vi "Main-revision2.vi"() -> ()   [LabVIEW 2020]
uses:
  Shared/GUI_Template/TCP subscription info cluster.ctl
  Controls/GUI controls/TabControl--Tab.ctl
  Controls/Loop_data--Cluster.ctl
  Controls/Graph_data--Cluster.ctl
  Controls/GUI controls/GUI_Flags.ctl
  Controls/Database Data.ctl
  Shared/MySQL/typedefs/mysql_authentication.ctl
  <userlib>/_OpenG.lib/array/array.llb/Filter 1D Array with Scalar (String)__ogtk.vi
  Shared/MySQL/Preset Query Enum.ctl
panel:
  out "TCP subscriptions info":T1
  out "StopQueue":refnum<queue>
  out "DataQueue":refnum<queue>
  out "error out":errorcluster
  out "error TCP Open":errorcluster
  out "error TCP  Write":errorcluster
  in  "Tab Control":enum32{"Home", "Settings", "Plot", "Save"}(tab)
  in  "Database Variable List":i32[](listbox)
  in  "Plotter ID (Simulate)":string
  out "Query":string
  in  "Add variables":bool
  out "Long Term Plot":cluster{timestamp[], dbl[]}[](graph)
  in  "Clear Graph":bool
  out "short Term Plot":cluster{timestamp[], dbl[]}[](graph) caption="Long Term Plot"
  in  "Stop":bool
  in  "Simulate":bool
  out "Data read by TCP":string[](array[string])
  out "appargs 2":string[](array[string])
  out "min Left":i16
  out "min Top":i16
  out "max Right":i16
  out "max Bottom":i16
  in  "Read INI File":bool
  in  "Configuration File Path":path=path "C:/Users/Priyanka/Documents/Plotter/Data/Plot Configuration.txt"
  out "Subscribe commands":string[](array[string])=["Wait>>Exposure,Gain", "Wait>>Exposure"]
  out "IP Addresses of interested  devices":string[](array[string])
  out "appended array":string[][](array[string])
  in  "reference out":refnum<vi>
  out "time to open ref":u32
  out "Device Infor from Database":string[][](array[string])
  in  "Plot":bool=TRUE
  in  "Settings":bool
  in  "Home":bool
  # "Settings"
  # "Plot"
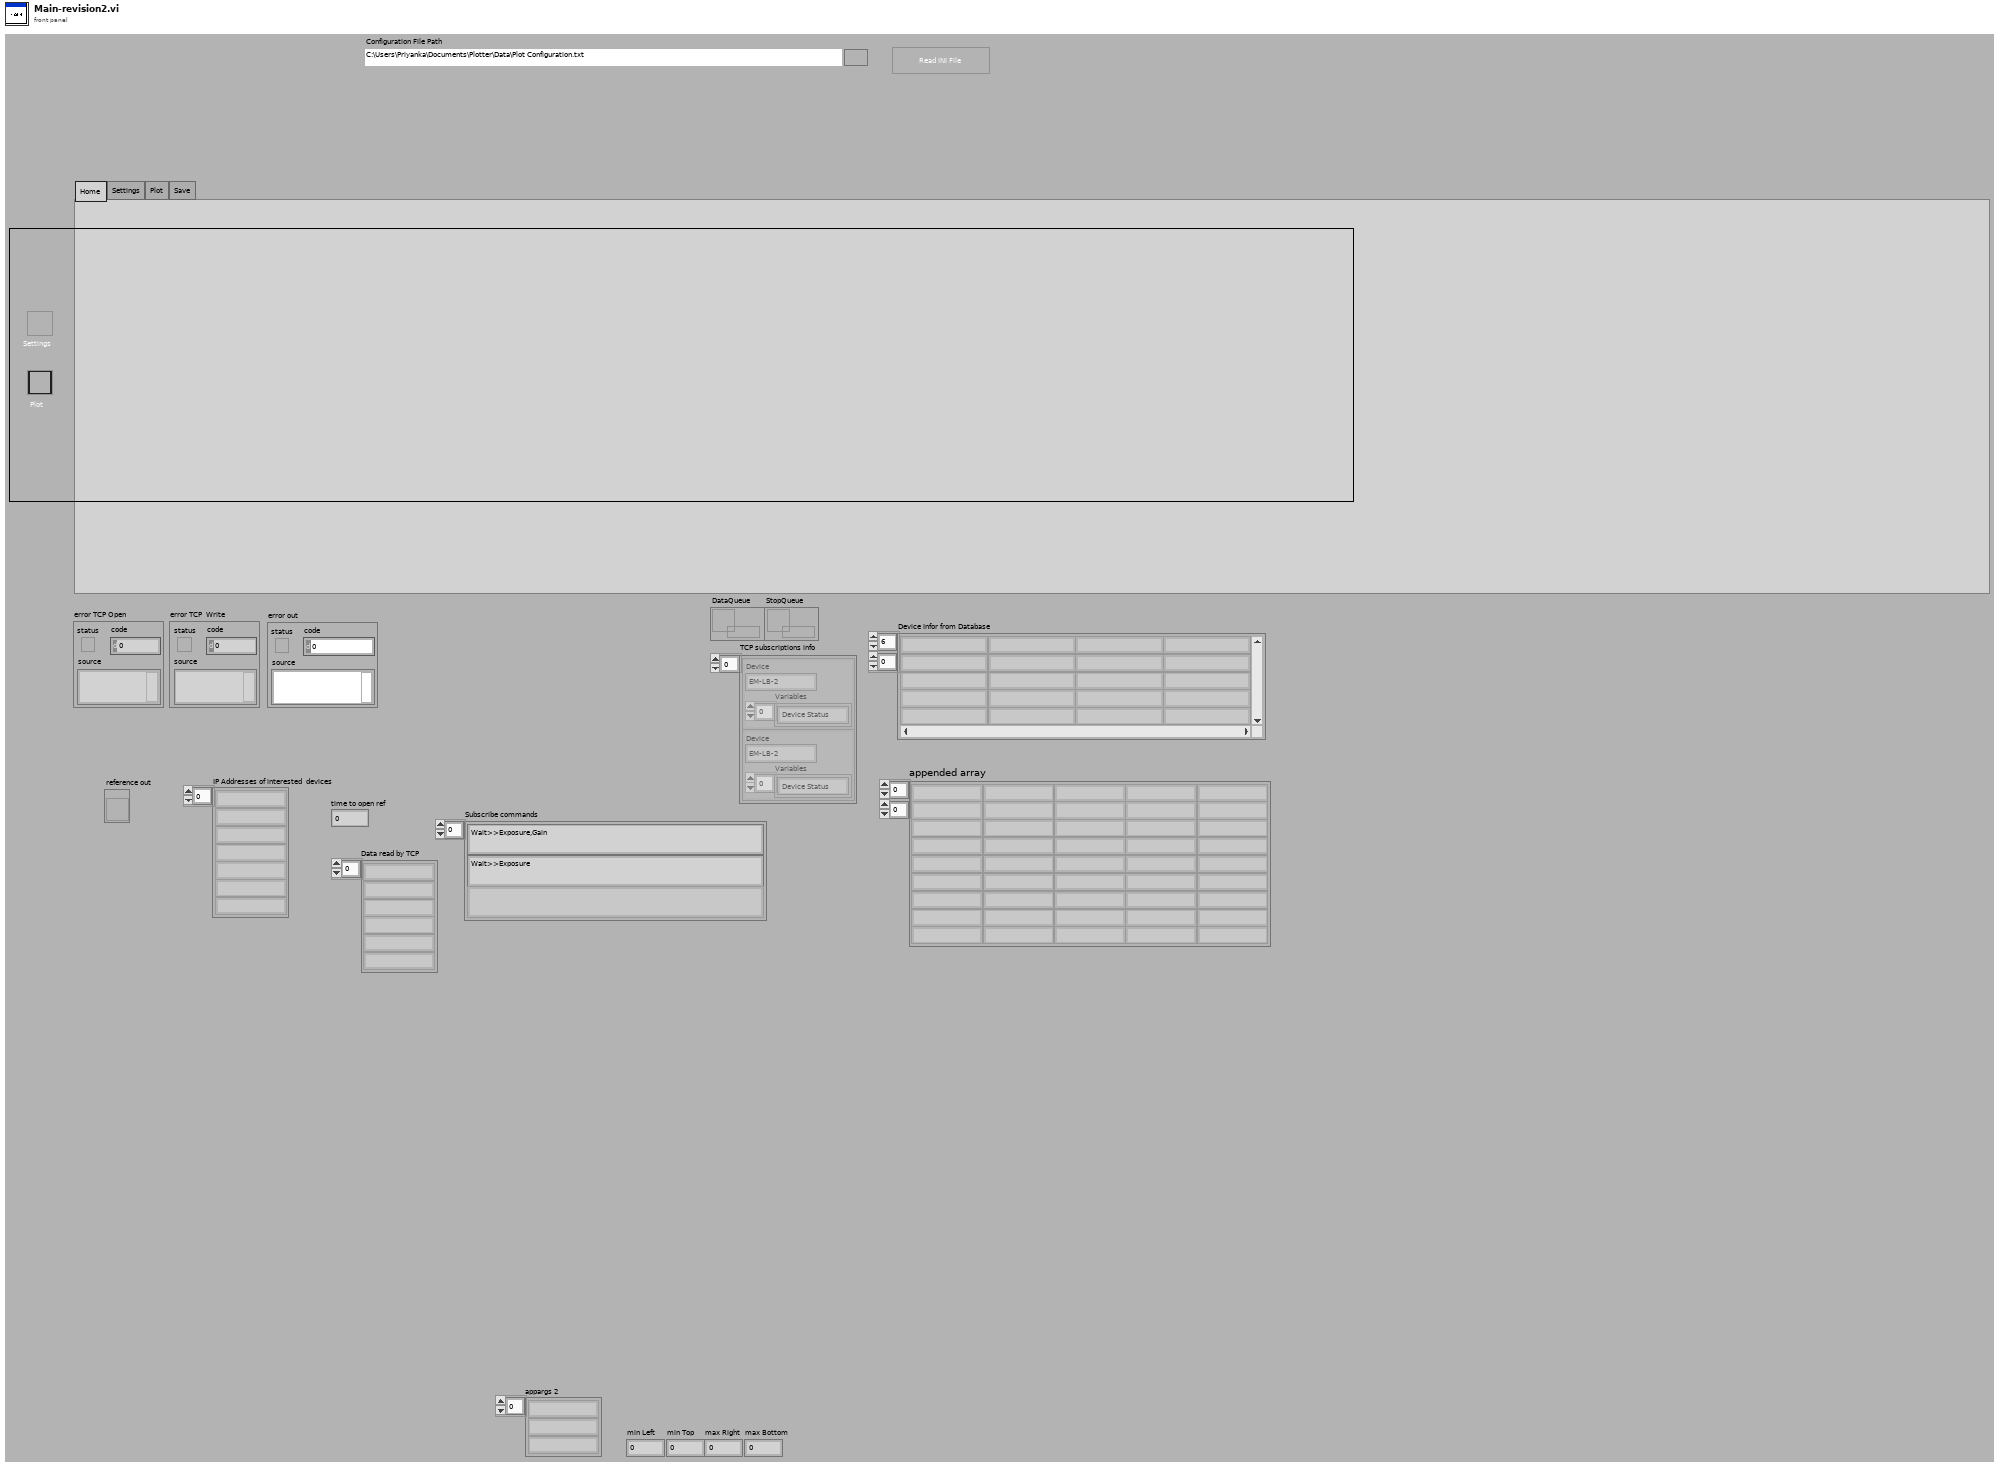
[diagram p1: front panel]
types:
  T1 = typedef "TCP subscription info cluster.ctl" = cluster{"Device":string, "Variables":string[]}[]
  T2 = typedef "LVAllMonitorsDisplayTypeDef.ctl" = cluster{"Bounds":cluster{"Left":i16, "Top":i16, "Right":i16, "Bottom":i16}, "Depth":i16}[]
  T3 = typedef "TabControl--Tab.ctl" = enum32{"Home", "Settings", "Plot", "Save"}
  T4 = cluster{"Selected Variables":string[][], "Data.TCP ports":refnum<k5>[]}
  T5 = enum32{"invalid app kind", "Development System", "Run Time System", "Student Edition", "Embedded LabVIEW", "Evaluation", "Custom"}
  T6 = typedef "Preset Query Enum.ctl" = enum16{"Get Locations", "Get all IPs and MACs", "Get classes", "Get expt variables to set at scanstart for particular device", "Get expt devices and variables with start values", "Get expt devices and variables (with data to get)", "Get expt devices with data to get", "Get Expt devices and GUIs", "Get all devices basic properties", "Get Virtual Devices Core Info", "Get Expt names", "Get experiment basic properties", "Get experiment alarm variables", "Get MC Ports", "Get device network comm port", "Get devicetype lvclass path", "Get basic device properties", "Get Init Order", "Get all setable variables of a device", "Get device variable aliases", "Get force values of all settable variables", "Get all variables of a devicetype", "Get all variables of a device", "Get plotter details", "Get Saved Scans", "Get Scan Info", "GetGeneralGUIs", "Get expt for plotter", "Get plotter IDs from expt", "Get all devices", "Get all Virtual Devices", "Get all aliases", "Get variable and device info for Virtual Device", "GetItemLocatorIP", "Get IPs for GUIs", "Get DeviceType from Device", "GetLocalPortRange", "GetDevicePresetVariables", "Get Device Configuration", "GetAllPresetNames", "GetAllConfigurationNames", "GetPresetDeviceNames", "GetDeviceAliases", "GetDevicesOfClass"}
  T7 = enum32{"Invalid", "Standard", "Closed", "Hidden", "Minimized", "Maximized"}
  T8 = typedef "Loop_data--Cluster.ctl" = cluster{"INI Data":string[][], "Currently selected items":i32[], "Selected Variables":string[][], "No of Selected Variables":i32, "Data":dbl[], "Simulate":bool, "Start":bool, "Legend Rows":i32, "Init":bool}
  T9 = typedef "Graph_data--Cluster.ctl" = cluster{"Graph Data Long":cluster{"Timestamp":timestamp[], "Data Array":dbl[]}[], "Graph Data Short":cluster{"Timestamp":timestamp[], "Data Array":dbl[]}[], "Short term plot":refnum<vi>, "Long term plot ":refnum<vi>, "ms timer value":u32}
  T10 = typedef "GUI_Flags.ctl" = cluster{"Start":bool, "Stop":bool, "Read INI File":bool, "Tab Control":enum32{"Home", "Settings", "Plot", "Save"}, "Settings":bool, "Home":bool, "Plot":bool}
  T11 = typedef "Database Data.ctl" = cluster{"SQL Server Info":cluster{"Port":u16, "IP Address":string, "Authentication":T12}, "Variables":string[], "Devices":string[], "Display Names (for variables)":string[], "Variable Data ID":string, "Variable display info":string[][], "Plotter ID":string, "Device space Variable":string[]}
  T12 = typedef "mysql_authentication.ctl" = cluster{"User":string, "Password":string, "Database":string}
  T13 = cluster{"Core":cluster{"Current VI Reference":refnum<vi>, "Close Panel on Exit?":bool}, "Data":T8, "Graph":T9, "reference out":refnum<vi>, "GUI controls":T10, "Database Data":T11, "TCP ports":refnum<k5>[]}
  T14 = cluster{"Current VI Reference":refnum<vi>, "Close Panel on Exit?":bool}
  T15 = cluster{"Port":u16, "IP Address":string, "Authentication":T12}
  T16 = cluster{"Timestamp":timestamp[], "Data Array":dbl[]}[]
  T17 = cluster{"Any timeouts?":bool, "tcp read times":u32[], "Errors":errorcluster[], "tcp Data parsed array":string[][]}
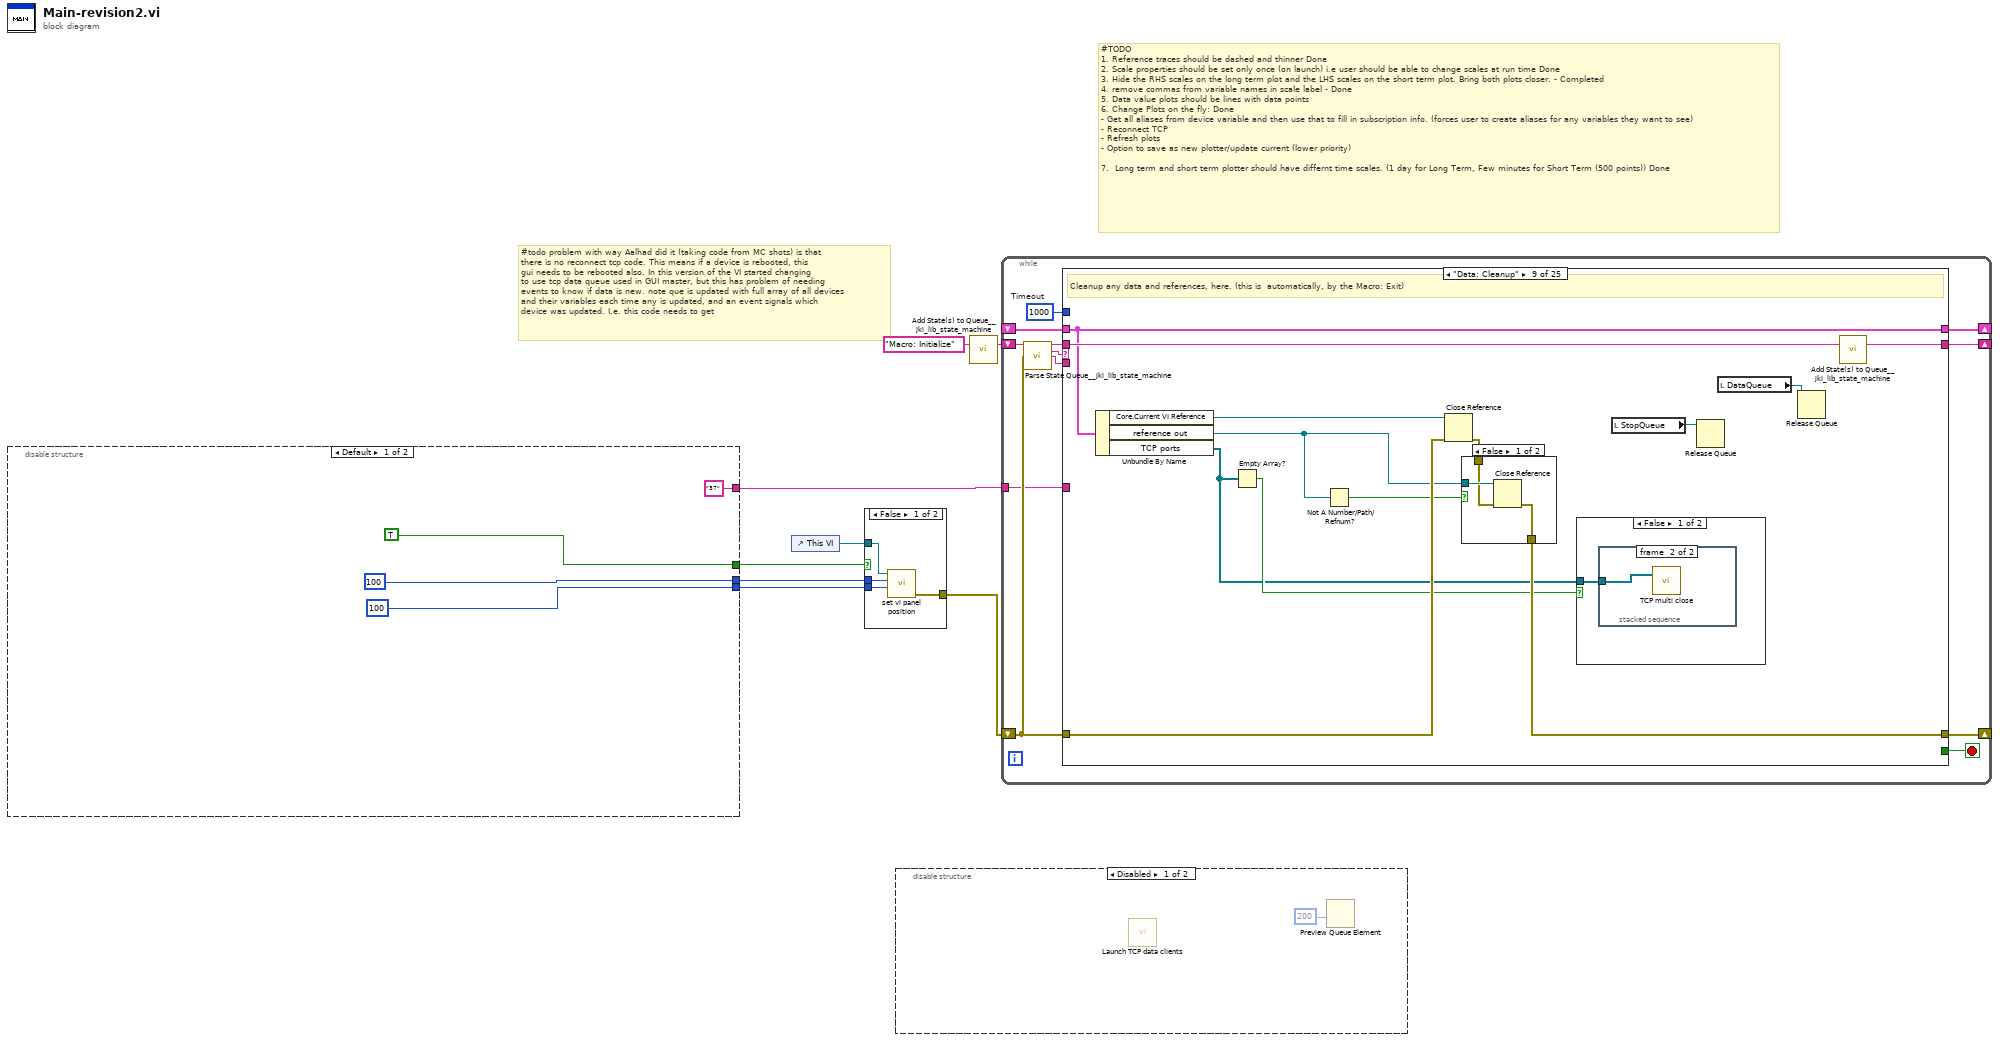
[diagram p0: block diagram]
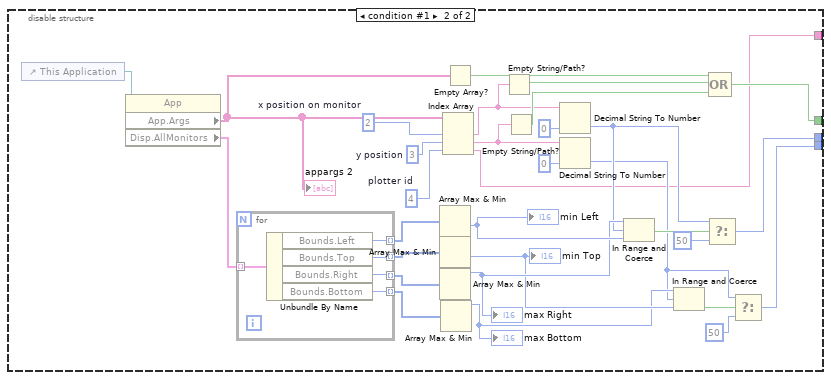
[diagram p4: hidden frame]
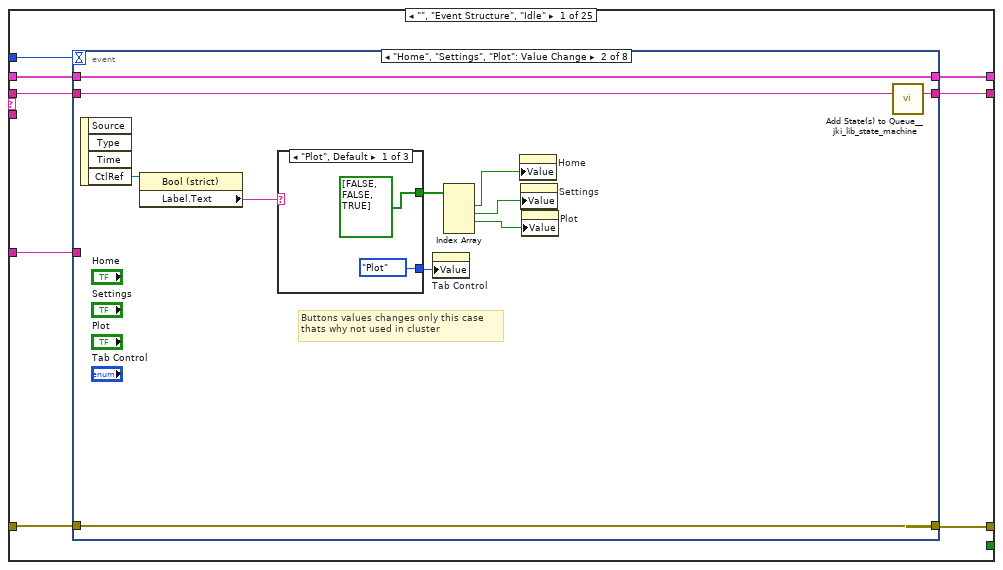
[diagram p5: hidden frame]
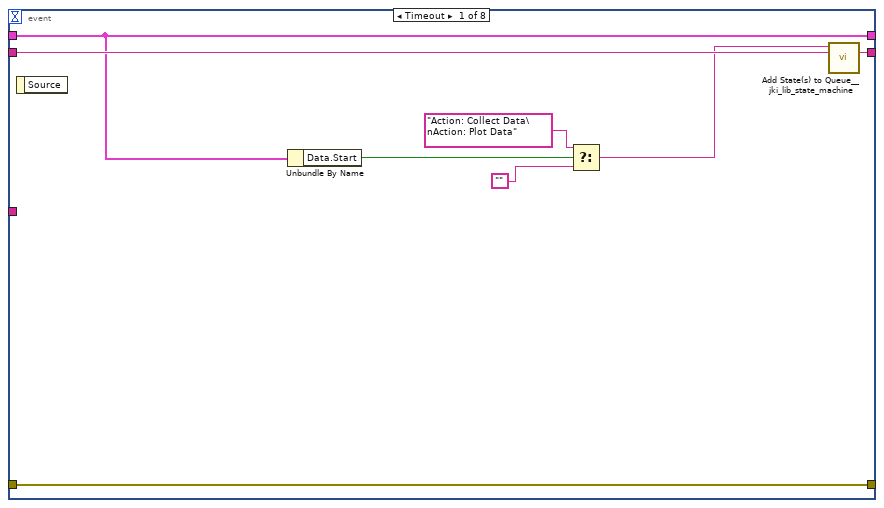
[diagram p6: hidden frame]
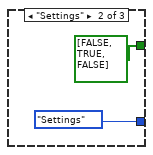
[diagram p7: hidden frame]
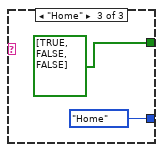
[diagram p8: hidden frame]
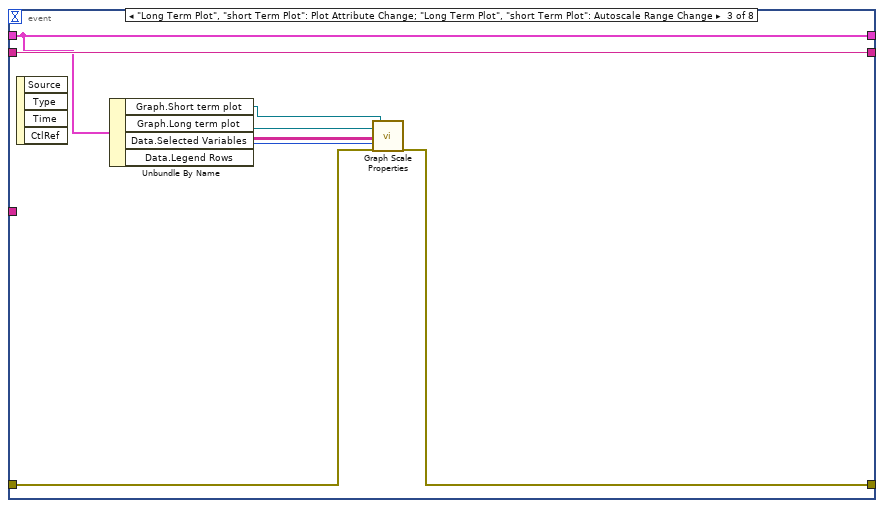
[diagram p9: hidden frame]
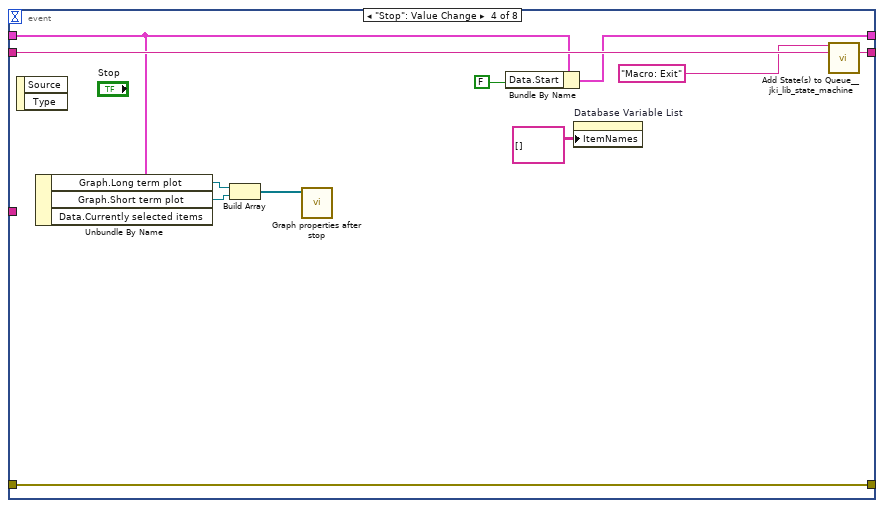
[diagram p10: hidden frame]
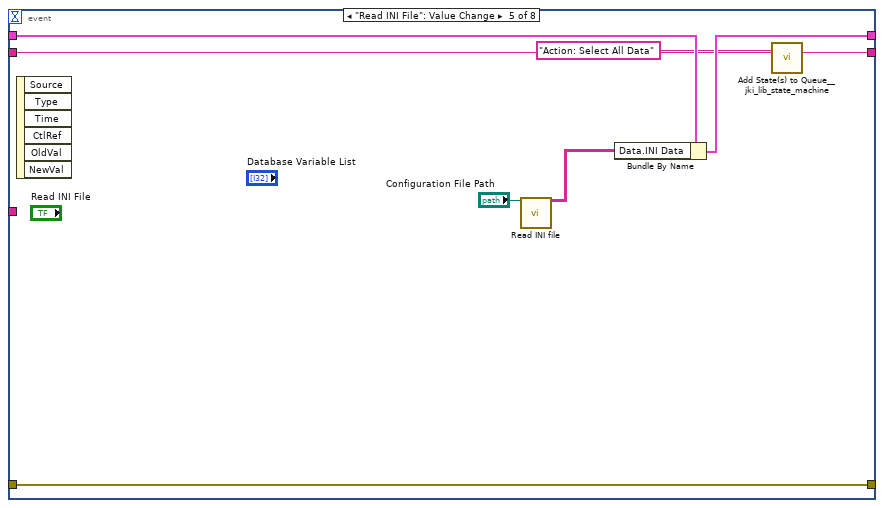
[diagram p11: hidden frame]
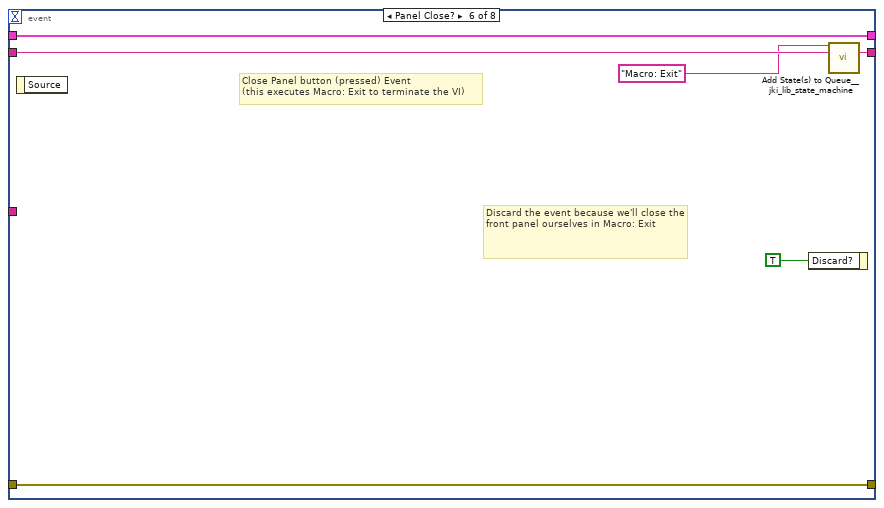
[diagram p12: hidden frame]
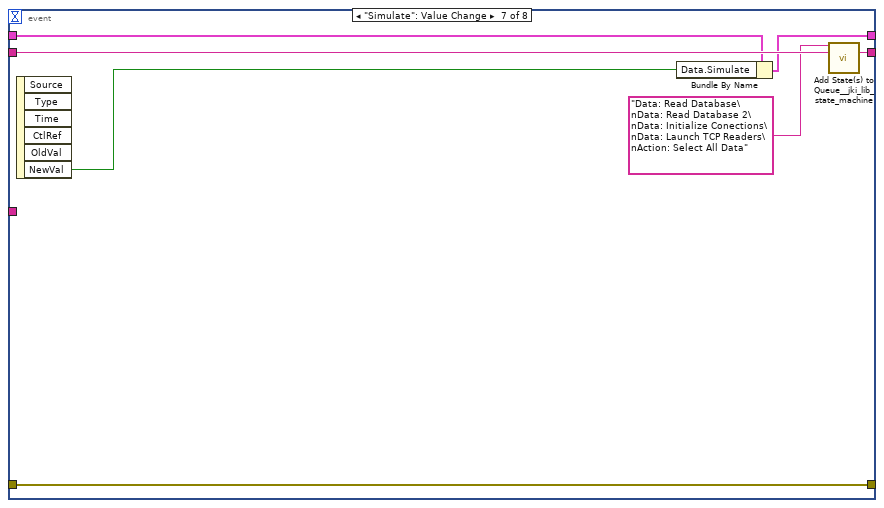
[diagram p13: hidden frame]
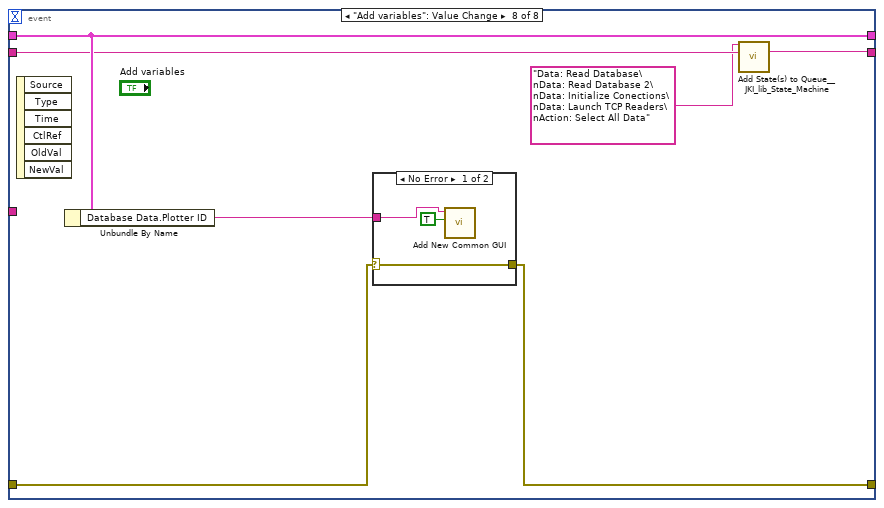
[diagram p14: hidden frame]
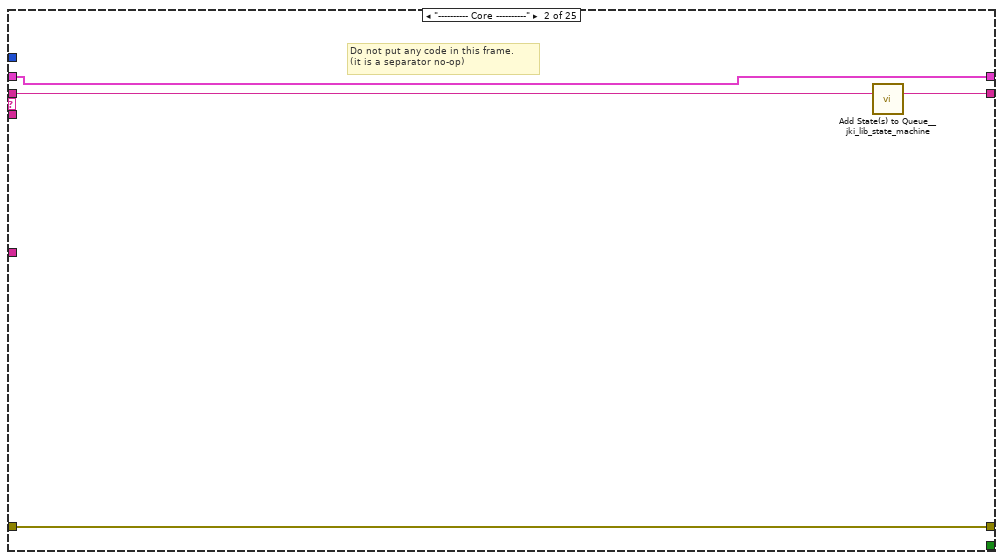
[diagram p16: hidden frame]
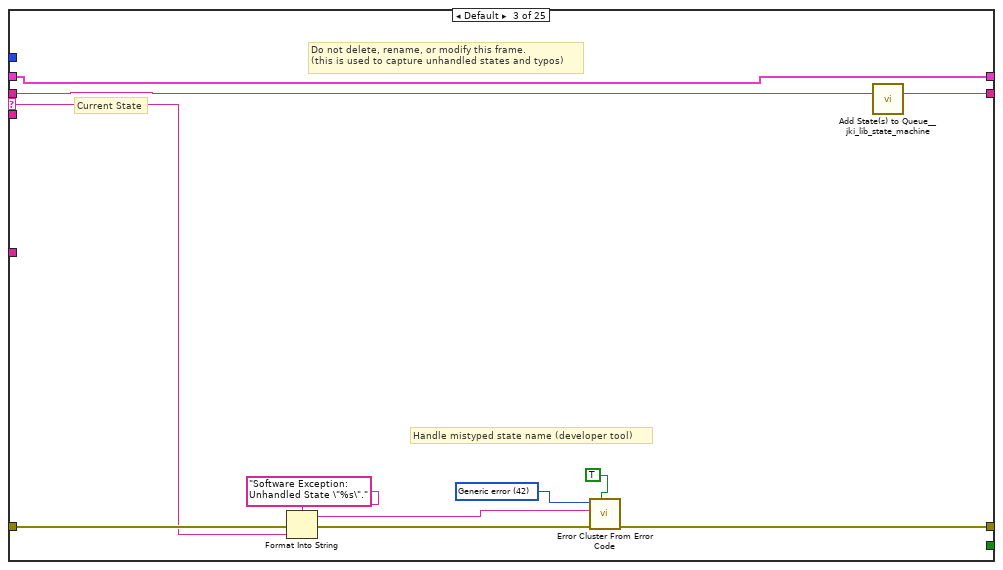
[diagram p17: hidden frame]
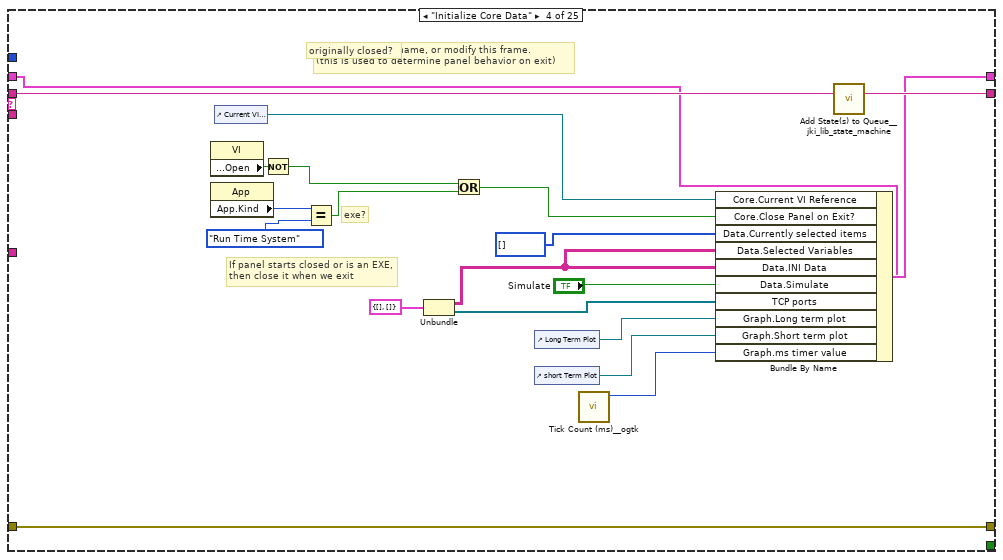
[diagram p18: hidden frame]
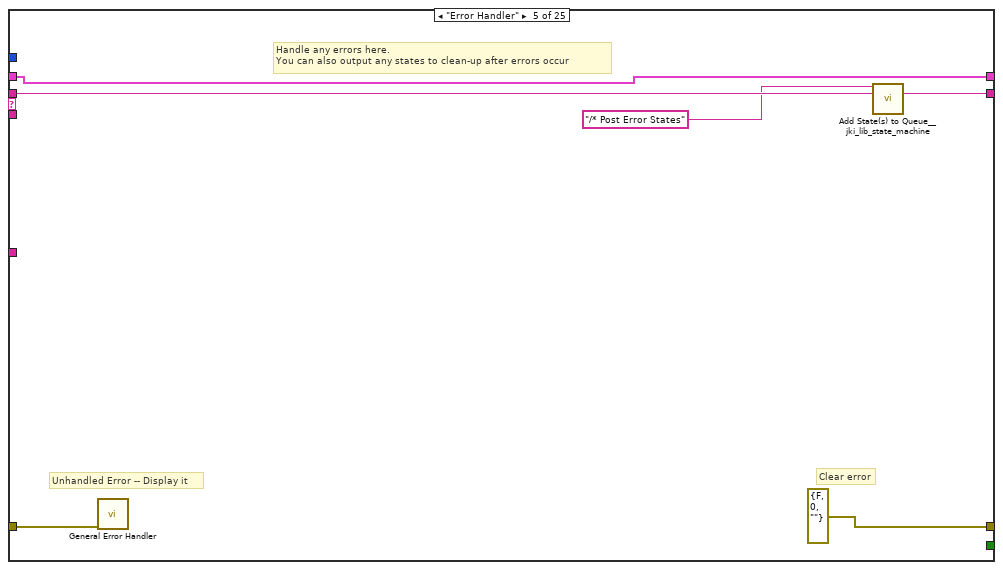
[diagram p19: hidden frame]
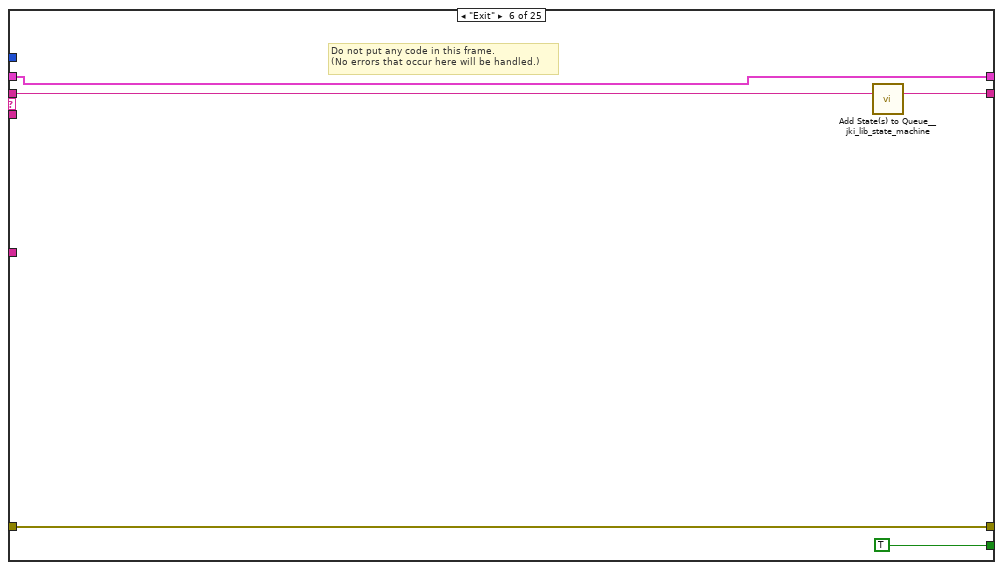
[diagram p20: hidden frame]
diagram:
  # "#todo problem with way Aalhad did it (taking code from MC shots) is that\nthere is no reconnect tcp code. This means if a device is rebooted, this\ngui needs to be rebooted also. In this version of the VI started changing\nto use tcp data queue used in GUI master, but this has problem of needing\nevents to know if data is new. note que is updated with full array of all devices\nand their variables each time any is updated, and an event signals which\ndevice was updated. I.e. this code needs to get"
  # "#TODO\n1. Reference traces should be dashed and thinner Done\n2. Scale properties should be set only once (on launch) i.e user should be able to change scales at run time Done\n3. Hide the RHS scales on the long term plot and the LHS scales on the short term plot. Bring both plots closer. - Completed\n4. remove commas from variable names in scale label - Done \n5. Data value plots should be lines with data points\n6. Change Plots on the fly: Done\n- Get all aliases from device variable and then use that to fill in subscription info. (forces user to create aliases for any variables they want to see)\n- Reconnect TCP\n- Refresh plots\n- Option to save as new plotter/update current (lower priority)\n\n7.  Long term and short term plotter should have differnt time scales. (1 day for Long Term, Few minutes for Short Term (500 points)) Done"
  n1 = disable-structure shown="Default" {
    disable-tunnel: [100 ("number") w27] -> w4
    disable-tunnel: [100 ("number") w22] -> w5
    disable-tunnel: [TRUE w17] -> w6
    disable-tunnel: ["37" w14] -> w1
    frame condition #0 (active) {
    }
    frame condition #1 {
      w15 = 4  # plotter id
      w42 = 3  # y position
      w43 = 2  # x position on monitor
      n2 = control-ref of="This Application"() -> (w16:refnum<vi>)
      n3 = property class="App"(reference=w16) -> ("App.Args"=w41:string[], "Disp.AllMonitors"=w36:T2)  [unwired: 1 in, 2 out]
      "appargs 2" <- w41
      n4 = for {
        tunnel: w36 -> [w48] mode=indexing
        tunnel: [w47] -> w37 mode=indexing
        tunnel: [w46] -> w38 mode=indexing
        tunnel: [w45] -> w39 mode=indexing
        tunnel: [w44] -> w40 mode=indexing
        n5 = Unbundle By Name(w48) -> ("Bounds.Left"=w47:i16, "Bounds.Top"=w46:i16, "Bounds.Right"=w45:i16, "Bounds.Bottom"=w44:i16)
      }
      n6 = Array Max & Min(array=w37) -> (min value=w35:i16)  [unwired: 3 out]
      "min Left" <- w35
      n7 = Array Max & Min(array=w38) -> (min value=w33:i16)  [unwired: 3 out]
      "min Top" <- w33
      n8 = Array Max & Min(array=w39) -> (max value=w34:i16)  [unwired: 3 out]
      "max Right" <- w34
      n9 = Array Max & Min(array=w40) -> (max value=w32:i16)  [unwired: 3 out]
      "max Bottom" <- w32
      n10 = Index Array(array=w41, index #1=w43, index #2=w42, index #3=w15) -> (element #1=w13:string, element #2=w21:string, element #3=w14:string)
      n11 = Empty Array?(array=w41) -> (empty?=w20:bool)
      n12 = Empty String/Path?(string/path=w13) -> (empty?=w19:bool)
      n13 = Empty String/Path?(string/path=w21) -> (empty?=w18:bool)
      n14 = Decimal String To Number(string=w13, default (0L)=i16 0 ("default (0 I32)")) -> (number=w28:i16)  [unwired: 1 in, 1 out]
      n15 = Decimal String To Number(string=w21, default (0L)=i16 0 ("default (0 I32)")) -> (number=w23:i16)  [unwired: 1 in, 1 out]
      n16 = In Range and Coerce(upper limit=w34, x=w28, lower limit=w35) -> (In Range?=w29:bool)  [unwired: 1 out]
      n17 = In Range and Coerce(upper limit=w32, x=w23, lower limit=w33) -> (In Range?=w24:bool)  [unwired: 1 out]
      n18 = Select(t=w28, s=w29, f=i16 50) -> (s? t:f=w27:i16)
      n19 = Compound Arithmetic op=OR(w20, w19, w18) -> (w17:bool)
      n20 = Select(t=w23, s=w24, f=i16 50) -> (s? t:f=w22:i16)
    }
  }
  n21 = control-ref of="This VI"() -> (w3:refnum<vi>)
  n22 = case shown="False" w6 {
    tunnel: w4 -> [w52 _]
    tunnel: w5 -> [w51 _]
    tunnel: w3 -> [w50 _]
    tunnel: [w49 _] -> w2
    frame False {
      n23 = call "set vi panel position.vi"("top"=w51, "left"=w52, "This VI"=w50) -> ("error out"=w49:errorcluster)  [unwired: 7 in, 1 out]
    }
    frame True {
    }
  }
  n24 = disable-structure shown="Disabled" {
    frame Disabled {
      n25 = call "Launch TCP data clients.vi"() -> ()  [unwired: 10 in, 2 out]
      n26 = Preview Queue Element(timeout in ms (-1)=200) -> ()  [unwired: 2 in, 4 out]
    }
    frame Enabled {
    }
  }
  n27 = call <vilib>:"Add State(s) to Queue__jki_lib_state_machine.vi"("State(s) in (\"\")"="Macro: Initialize") -> ("States Out"=w8:string)  [unwired: 14 in]
  n28 = while {
    shift-right: [w59] -> _
    shift-left: _ -> [w58]
    shift-right: [w62] -> _
    shift-left: w2 -> [w56]
    shift-right: [w61] -> _
    shift-left: w8 -> [w63]
    tunnel: w1 -> [w54]
    stop <- w60 stop-if-true
    w57 = 1000  # Timeout
    n29 = call <vilib>:"Parse State Queue__jki_lib_state_machine.vi"("State Queue"=w63, "Error In (no error)"=w56) -> ("Remaining States"=w65:string, "Current State"=w55:string, "Arguments"=w64:string)  [unwired: 11 in]
    n30 = case shown="\"Data: Cleanup\"" w55 {
      selector: w55 -> [_ _ w154 _ _ _ _ _ _ _ _ _ _ _ _ _ _ _ _ _ _ _ _ _ _]
      tunnel: w65 -> [w73 w153 w158 w184 w190 w195 w199 w210 w223 w252 w285 w299 w335 w371 w381 w387 w398 w424 w431 w441 w445 w449 w481 w507 w557]
      tunnel: w64 -> [_ _ _ _ _ _ _ _ _ _ _ _ _ _ _ w382 w392 _ _ _ _ _ _ _ _]
      tunnel: w58 -> [w71 w150 w156 w175 w187 w193 w196 _ w219 w237 w279 w296 w329 w368 w372 w385 w394 w421 w426 w438 w442 w451 w476 w501 w553]
      tunnel: [w70 w151 w160 w181 errorcluster {"status"=FALSE, "code"=0, "source"=""} ("error out") w192 w197 w207 w217 w250 w282 w291 w330 w369 w379 w383 w395 w422 w428 w439 w443 w457 w479 w502 w549] -> w62
      tunnel: w56 -> [w69 w151 w159 w181 w186 w192 w197 w207 w220 w250 w283 w292 w331 w369 w379 w384 w396 w422 w429 w439 w443 w457 w479 w503 w541]
      tunnel: [w72 w152 w157 w183 w189 w194 w198 w209 w222 w251 w284 w298 w334 w370 w380 w386 w397 w423 w430 w440 w444 w448 w480 w506 w556] -> w61
      tunnel: [_ _ _ _ _ TRUE _ _ _ _ _ _ _ _ _ _ _ _ _ _ _ _ _ _ _] -> w60
      tunnel: [w68 w150 w156 w182 w187 w193 w196 w208 w219 w249 w281 w295 w327 w368 w372 w385 w394 w421 w426 w438 w442 w450 w477 w500 w555] -> w59
      tunnel: w57 -> [w67 _ _ _ _ _ _ _ _ _ _ _ _ _ _ _ _ _ _ _ _ _ _ _ _]
      tunnel: w54 -> [w66 _ _ _ _ _ _ _ _ w234 _ _ _ _ _ _ _ _ _ _ _ _ _ _ _]
      frame "", "Event Structure", "Idle" {
        n31 = event shown="[1] \"Home\", \"Settings\", \"Plot\": Value Change" {
          selector: _ -> [_ _ _ _ _ _ _ _]
          dyn-events: _ -> [_ _ _ _ _ _ _ _]
          timeout: w67 -> [_ _ _ _ _ _ _ _]
          tunnel: w73 -> [w81 w92 w106 w117 w120 w131 w138 w143]
          tunnel: [w80 w91 w106 w116 w119 w130 w137 w142] -> w72
          tunnel: w71 -> [w77 w86 w105 w111 w122 w128 w135 w145]
          tunnel: [w79 w90 w101 w115 w125 w129 w136 w139] -> w70
          tunnel: w69 -> [w79 w90 w102 w115 w125 w129 w136 w140]
          tunnel: [w77 w86 w105 w113 w121 w128 w134 w145] -> w68
          tunnel: w66 -> [_ _ _ _ _ _ _ _]
          event Timeout {
            n32 = event-data() -> ()  [unwired: 1 in, 1 out]
            n33 = Unbundle By Name(w77) -> ("Data.Start"=w76:bool)
            n34 = Select(t="Action: Collect Data\nAction: Plot Data" ("f"), s=w76, f="") -> (s? t:f=w78:string)
            n35 = call <vilib>:"Add State(s) to Queue__jki_lib_state_machine.vi"("State(s) in Front (\"\")"=w78, "State(s) in (\"\")"=w81) -> ("States Out"=w80:string)  [unwired: 13 in]
          }
          event "Home", "Settings", "Plot": Value Change {
            # "Buttons values changes only this case \nthats why not used in cluster"
            n36 = event-data() -> ("CtlRef"=w89:refnum<vi>)  [unwired: 1 in, 3 out]
            n37 = property class="Bool (strict)"(reference=w89) -> ("Label.Text"=w88:string)  [unwired: 1 in, 2 out]
            n38 = case shown="\"Plot\", Default" w88 {
              tunnel: [TabControl--Tab."Plot" ("Tab Control") TabControl--Tab."Settings" ("Tab Control") TabControl--Tab."Home" ("Tab Control")] -> w82
              tunnel: [bool[] [FALSE, FALSE, TRUE] bool[] [FALSE, TRUE, FALSE] bool[] [TRUE, FALSE, FALSE]] -> w87
              frame "Plot", Default {
              }
              frame "Settings" {
              }
              frame "Home" {
              }
            }
            n39 = property on="Tab Control" class="TabCtl (strict)"("Value"=w82) -> ()  [unwired: 2 in, 2 out]
            n40 = Index Array(array=w87) -> (element #1=w85:bool, element #2=w84:bool, element #3=w83:bool)  [unwired: 4 in, 1 out]
            n41 = property on="Home" class="Bool (strict)"("Value"=w85) -> ()  [unwired: 2 in, 2 out]
            n42 = property on="Settings" class="Bool (strict)"("Value"=w84) -> ()  [unwired: 2 in, 2 out]
            n43 = property on="Plot" class="Bool (strict)"("Value"=w83) -> ()  [unwired: 2 in, 2 out]
            n44 = call <vilib>:"Add State(s) to Queue__jki_lib_state_machine.vi"("State(s) in (\"\")"=w92) -> ("States Out"=w91:string)  [unwired: 14 in]
          }
          event "Long Term Plot", "short Term Plot": Plot Attribute Change; "Long Term Plot", "short Term Plot": Autoscale Range Change {
            n45 = event-data() -> ()  [unwired: 1 in, 4 out]
            n46 = Unbundle By Name(w105) -> ("Graph.Short term plot"=w103:refnum<vi>, "Graph.Long term plot"=w99:refnum<vi>, "Data.Selected Variables"=w104:string[][], "Data.Legend Rows"=w100:i32)
            n47 = call "Graph Scale Properties.vi"("Long term plot"=w99, "Selected Variables"=w104, "Legend Rows"=w100, "error in (no error)"=w102, "Short term graph"=w103) -> ("error out"=w101:errorcluster)  [unwired: 14 in]
          }
          event "Stop": Value Change {
            n48 = event-data() -> ()  [unwired: 1 in, 2 out]
            n49 = Unbundle By Name(w111) -> ("Graph.Long term plot"=w108:refnum<vi>, "Graph.Short term plot"=w107:refnum<vi>)  [unwired: 1 out]
            n50 = Build Array(w108, w107) -> (w109:refnum<vi>[])
            n51 = call "Graph properties after stop.vi"("Array"=w109) -> ()  [unwired: 11 in]
            n52 = Bundle By Name(cluster=w111, "Data.Start"=FALSE) -> (w113:T13)
            n53 = property on="Database Variable List" class="MCListbox (strict)"("ItemNames"=string[][] [] ("Item Names")) -> ()  [unwired: 2 in, 2 out]
            n54 = call <vilib>:"Add State(s) to Queue__jki_lib_state_machine.vi"("State(s) in Front (\"\")"="Macro: Exit", "State(s) in (\"\")"=w117) -> ("States Out"=w116:string)  [unwired: 13 in]
          }
          event "Read INI File": Value Change {
            n55 = event-data() -> ()  [unwired: 1 in, 6 out]
            n56 = call "Read INI file.vi"("Path"="Configuration File Path") -> ("Data"=w123:string[][])  [unwired: 9 in, 5 out]
            n57 = Bundle By Name(cluster=w122, "Data.INI Data"=w123) -> (w121:T13)
            n58 = call <vilib>:"Add State(s) to Queue__jki_lib_state_machine.vi"("State(s) in Front (\"\")"="Action: Select All Data" ("State(s) in Front (\"\")"), "State(s) in (\"\")"=w120) -> ("States Out"=w119:string)  [unwired: 13 in]
          }
          event Panel Close? {
            # "Discard the event because we'll close the front panel ourselves in Macro: Exit"
            # "Close Panel button (pressed) Event\n(this executes Macro: Exit to terminate the VI)"
            n59 = event-data() -> ()  [unwired: 1 in, 1 out]
            n60 = event-data("Discard?"=TRUE) -> ()  [unwired: 1 in, 1 out]
            n61 = call <vilib>:"Add State(s) to Queue__jki_lib_state_machine.vi"("State(s) in Front (\"\")"="Macro: Exit", "State(s) in (\"\")"=w131) -> ("States Out"=w130:string)  [unwired: 13 in]
          }
          event "Simulate": Value Change {
            n62 = event-data() -> ("NewVal"=w133:bool)  [unwired: 1 in, 5 out]
            n63 = Bundle By Name(cluster=w135, "Data.Simulate"=w133) -> (w134:T13)
            n64 = call <vilib>:"Add State(s) to Queue__jki_lib_state_machine.vi"("State(s) in Front (\"\")"="Data: Read Database\nData: Read Database 2\nData: Initialize Conections\nData: Launch TCP Readers\nAction: Select All Data" ("State(s) in Front (\"\")"), "State(s) in (\"\")"=w138) -> ("States Out"=w137:string)  [unwired: 13 in]
          }
          event "Add variables": Value Change {
            n65 = event-data() -> ()  [unwired: 1 in, 6 out]
            n66 = Unbundle By Name(w145) -> ("Database Data.Plotter ID"=w144:string)
            n67 = case shown="No Error" w140 {
              selector: w140 -> [w146 w149]
              tunnel: w144 -> [w147 _]
              tunnel: [w146 w149] -> w139
              frame No Error {
                n68 = call "Add New Common GUI.vi"("With Alias"=TRUE, "Plotter ID"=w147) -> ()  [unwired: 10 in]
              }
              frame Error {
              }
            }
            n69 = call <vilib>:"Add State(s) to Queue__JKI_lib_State_Machine.vi"("State(s) in Front (\"\")"="Data: Read Database\nData: Read Database 2\nData: Initialize Conections\nData: Launch TCP Readers\nAction: Select All Data", "State(s) in (\"\")"=w143) -> ("States Out"=w142:string)  [unwired: 13 in]
          }
        }
      }
      frame "---------- Core ----------" {
        # "Do not put any code in this frame.\n(it is a separator no-op)"
        n70 = call <vilib>:"Add State(s) to Queue__jki_lib_state_machine.vi"("State(s) in (\"\")"=w153) -> ("States Out"=w152:string)  [unwired: 14 in]
      }
      frame Default {
        w163 = 42 items=["No error", "Argument error", "Memory is full", "Out of zone", "End of file", "File already open", "Generic file I/O error", "File not found", "File permission error", "Disk is full", "Duplicate path", "Too many files open", "System feature not enabled", "Resource file not found", "Cannot add resource", "Resource not found", "Image not found", "Image memory error", "Pen does not exist", "Config type invalid", "Config token not found", "Config parse error", "Config memory error", "Bad external code format", "Bad external code offset", "External code not present", "Null window", "Destroy window error", "Null menu", "Print aborted", "Bad print record", "Print driver error", "Windows error during printing", "Memory error during printing", "Print dialog error", "Generic print error", "Invalid device refnum", "Device not found", "Device parameter error", "Device unit error", "Cannot open device", "Device call aborted", "Generic error", "Cancelled by user", "Object ID too low", "Object ID too high", "Object not in heap", "Unknown heap", "Unknown object (invalid DefProc)", "Unknown object (DefProc not in table)", "Message out of range", "Invalid (null) method", "Unknown message", "Manager call not supported", "Bad address", "Network operation in progress", "Network operation timed out", "Connection is busy", "Network attribute not supported", "Network error", "Address in use", "System out of memory", "Connection aborted", "Connection refused", "Not connected", "Already connected", "Connection closed", "Initialization error (interapplication manager)", "Bad occurrence", "Wait on unbound occurrence handler", "Occurrence queue overflow", "Datalog type conflict", "Unused", "Unrecognized type (interapplication manager)", "Memory corrupt", "Failed to make temporary DLL", "Old CIN version", "Drag socket not found", "Failed to load drop-object", "Failed to register OLE object", "Failed to release OLE object", "Format specifier type mismatch", "Unknown format specifier", "Too few format specifiers", "Too many format specifiers", "Scan failed", "Newer CIN version", "Error converting to variant", "Runtime menu error", "Password tampered", "Variant attribute not found", "Incompatible variant data type", "Event data is not available", "Event Store is not present", "Occurrence is not found", "Event Queue is not created", "Event info is not available", "Refnum passed is NULL", "Error retrieving Class GUID", "Error retrieving CoClass GUID", "Error retrieving TypeLib GUID.", "Bad built application magic bytes.", "Specific driver is different from the specific driver associated with the Logical Name.", "There is no session opened to the class driver.", "Max Error", "MAX - Error with config objects", "MAX - Error loading configuration", "MAX - Group not supported"]
        # "Current State"
        # "Do not delete, rename, or modify this frame.\n(this is used to capture unhandled states and typos)"
        # "Handle mistyped state name (developer tool)"
        n71 = Format Into String(format string="Software Exception: Unhandled State \"%s\"." ("message"), error in=w159, w154) -> (resulting string=w162:string, error out=w161:errorcluster)  [unwired: 1 in]
        n72 = call <vilib>:"Error Cluster From Error Code.vi"("show call chain? (False)"=TRUE, "error in (no error)"=w161, "error message (\"\")"=w162, "error code (0)"=w163) -> ("error out"=w160:errorcluster)  [unwired: 5 in]
        n73 = call <vilib>:"Add State(s) to Queue__jki_lib_state_machine.vi"("State(s) in (\"\")"=w158) -> ("States Out"=w157:string)  [unwired: 14 in]
      }
      frame "Initialize Core Data" {
        # "Do not delete, rename, or modify this frame.\n(this is used to determine panel behavior on exit)"
        # "originally closed?"
        # "exe?"
        # "If panel starts closed or is an EXE, then close it when we exit"
        n74 = property class="VI"() -> ("Front Panel.Open"=w180:bool)  [unwired: 2 in, 2 out]
        n75 = property class="App"() -> ("App.Kind"=w179:T5)  [unwired: 2 in, 2 out]
        n76 = control-ref of="Current VI Reference"() -> (w173:refnum<vi>)
        n77 = Not(x=w180) -> (.not. x?=w177:bool)
        n78 = Equal?(x=w179, y=T5."Run Time System" ("Application:Kind")) -> (x = y?=w176:bool)
        n79 = Unbundle(T4 {"Selected Variables"=[], "Data.TCP ports"=[]}) -> ("Selected Variables"=w167:string[][], "Data.TCP ports"=w166:refnum<k5>[])
        n80 = Or(x=w177, y=w176) -> (x .or. y?=w174:bool)
        n81 = control-ref of="Long Term Plot"() -> (w170:refnum<vi>)
        n82 = control-ref of="short Term Plot"() -> (w169:refnum<vi>)
        n83 = call <userlib>:"Tick Count (ms)__ogtk.vi"() -> ("millisecond timer value"=w165:u32)  [unwired: 10 in, 1 out]
        n84 = Bundle By Name(cluster=w175, "Core.Current VI Reference"=w173, "Core.Close Panel on Exit?"=w174, "Data.Currently selected items"=i32[] [], "Data.Selected Variables"=w167, "Data.INI Data"=w167, "Data.Simulate"="Simulate", "TCP ports"=w166, "Graph.Long term plot"=w170, "Graph.Short term plot"=w169, "Graph.ms timer value"=w165) -> (w182:T13)
        n85 = call <vilib>:"Add State(s) to Queue__jki_lib_state_machine.vi"("State(s) in (\"\")"=w184) -> ("States Out"=w183:string)  [unwired: 14 in]
      }
      frame "Error Handler" {
        # "Unhandled Error -- Display it"
        # "Handle any errors here.\nYou can also output any states to clean-up after errors occur"
        # "Clear error"
        n86 = call <vilib>:"General Error Handler.vi"("error in (no error)"=w186) -> ()  [unwired: 10 in, 5 out]
        n87 = call <vilib>:"Add State(s) to Queue__jki_lib_state_machine.vi"("State(s) in Front (\"\")"="/* Post Error States", "State(s) in (\"\")"=w190) -> ("States Out"=w189:string)  [unwired: 13 in]
      }
      frame "Exit" {
        # "Do not put any code in this frame.\n(No errors that occur here will be handled.)"
        n88 = call <vilib>:"Add State(s) to Queue__jki_lib_state_machine.vi"("State(s) in (\"\")"=w195) -> ("States Out"=w194:string)  [unwired: 14 in]
      }
      frame "---------- Data ----------" {
        # "Do not put any code in this frame.\n(It is a separator no-op. You can make a copy of this frame to create a new Data frame)"
        n89 = call <vilib>:"Add State(s) to Queue__jki_lib_state_machine.vi"("State(s) in (\"\")"=w199) -> ("States Out"=w198:string)  [unwired: 14 in]
      }
      frame "Data: Initialize" {
        w200 = refnum<k5>[] []  # TCP ports
        w201 = T11 {"SQL Server Info"={"Port"=0, "IP Address"="", "Authentication"={"User"="", "Password"="", "Database"=""}}, "Variables"=[], "Devices"=[], "Display Names (for variables)"=[], "Variable Data ID"="", "Variable display info"=[], "Plotter ID"="", "Device space Variable"=[]}  # Database Data
        w202 = T10 {"Start"=FALSE, "Stop"=TRUE, "Read INI File"=TRUE, "Tab Control"=enum."Plot", "Settings"=FALSE, "Home"=FALSE, "Plot"=TRUE}  # GUI controls
        w203 = T9 {"Graph Data Long"=[], "Graph Data Short"=[], "Short term plot"=refnum, "Long term plot "=refnum, "ms timer value"=0}  # Graph
        w205 = T8 {"INI Data"=[], "Currently selected items"=[], "Selected Variables"=[], "No of Selected Variables"=0, "Data"=[], "Simulate"=FALSE, "Start"=FALSE, "Legend Rows"=0, "Init"=FALSE}  # Data
        w206 = T14 {"Current VI Reference"=refnum, "Close Panel on Exit?"=FALSE}  # Core
        n90 = Bundle("Core"=w206, "Data"=w205, "Graph"=w203, "reference out"="reference out", "GUI controls"=w202, "Database Data"=w201, "TCP ports"=w200) -> (w208:T13)  [unwired: 1 in]
        n91 = call <vilib>:"Add State(s) to Queue__jki_lib_state_machine.vi"("State(s) in (\"\")"=w210) -> ("States Out"=w209:string)  [unwired: 14 in]
      }
      frame "Data: Cleanup" {
        # "Cleanup any data and references, here. (this is  automatically, by the Macro: Exit)"
        n92 = Unbundle By Name(w219) -> ("Core.Current VI Reference"=w221:refnum<vi>, "reference out"=w216:refnum<vi>, "TCP ports"=w213:refnum<k5>[])
        n93 = Empty Array?(array=w213) -> (empty?=w214:bool)
        n94 = Not A Number/Path/Refnum?(number/path/refnum=w216) -> (NaN/Path/Refnum?=w215:bool)
        n95 = Close Reference(reference=w221, error in (no error)=w220) -> (error out=w218:errorcluster)
        n96 = case shown="False" w215 {
          tunnel: w216 -> [w231 _]
          tunnel: w218 -> [w230 w232]
          tunnel: [w229 w232] -> w217
          frame False {
            n97 = Close Reference(reference=w231, error in (no error)=w230) -> (error out=w229:errorcluster)
          }
          frame True {
          }
        }
        n98 = case shown="False" w214 {
          tunnel: w213 -> [w224 _]
          frame False {
            n99 = stacked-sequence {
              tunnel: w224 -> [w225 w228]
              frame #0 {
                n100 = for {
                  tunnel: w225 -> [w227] mode=indexing
                  n101 = call "clearTCPBufferSerial.vi"("connection ID in"=w227) -> ("error out"=w226:errorcluster)  [unwired: 9 in, 1 out]
                  n102 = call <vilib>:"Clear Errors.vi"("error in (no error)"=w226) -> ()  [unwired: 5 in, 2 out]
                }
              }
              frame #1 {
                n103 = call "TCP multi close.vi"("TCP Ports"=w228) -> ()  [unwired: 2 in, 1 out]
              }
            }
          }
          frame True {
          }
        }
        n104 = local read "StopQueue"() -> (w212:refnum<queue>)
        n105 = Release Queue(queue=w212) -> ()  [unwired: 2 in, 3 out]
        n106 = local read "DataQueue"() -> (w211:refnum<queue>)
        n107 = Release Queue(queue=w211) -> ()  [unwired: 2 in, 3 out]
        n108 = call <vilib>:"Add State(s) to Queue__jki_lib_state_machine.vi"("State(s) in (\"\")"=w223) -> ("States Out"=w222:string)  [unwired: 14 in]
      }
      frame "Data: Read Database" {
        w240 = 0 ("disabled index (col)")
        # "Get Device, Variable Names and Display Names from commongui Table"
        n109 = Unbundle By Name(w237) -> ("Data.Simulate"=w236:bool)
        n110 = Select(t="Plotter ID (Simulate)", s=w236, f=w234) -> (s? t:f=w233:string)
        n111 = Concatenate Strings("SELECT variablesid FROM commongui WHERE id ='", w233, "'" ("string")) -> (w241:string)
        "Query" <- w241
        n112 = call "SQL Server Info.vi"() -> ("SQL Server Info"=w248:T15)
        n113 = call "SQL Query.vi"("error in (no error)"=w250, "SQL Server Info"=w248, "Query"=w241) -> ("data"=w239:string[][])  [unwired: 7 in, 1 out]
        n114 = Empty Array?(array=w239) -> (empty?=w238:bool)
        n115 = case shown="True" w238 {
          tunnel: w233 -> [_ w253]
          frame False {
          }
          frame True {
            n116 = Concatenate Strings("Please Check Plotter ID [" ("string"), w253, "] Plotter ID should match with id from commongui Table in Database." ("message")) -> (w254:string)
            n117 = One Button Dialog(message=w254, button name ("OK")="OK") -> ()  [unwired: 1 out]
          }
        }
        n118 = Index Array(array=w239, index (row)=w240, index (col)=w240) -> (element=w247:string)
        n119 = call "Get Device List.vi"("SQL Server Info"=w248, "userID"=w247) -> ("Display Names"=w244:string[], "Variables"=w245:string[], "Devices"=w246:string[])  [unwired: 7 in]
        n120 = Bundle By Name(cluster=w237, "Database Data.SQL Server Info"=w248, "Database Data.Variable Data ID"=w247, "Database Data.Devices"=w246, "Database Data.Variables"=w245, "Database Data.Display Names (for variables)"=w244, "Database Data.Plotter ID"=w233) -> (w249:T13)
        n121 = call <vilib>:"Add State(s) to Queue__jki_lib_state_machine.vi"("State(s) in (\"\")"=w252) -> ("States Out"=w251:string)  [unwired: 14 in]
      }
      frame "Data: Read Database 2" {
        # "Get variable data from commongui_variables Table"
        n122 = Unbundle By Name(w279) -> ("Database Data.Devices"=w266:string[], "Database Data.Variables"=w265:string[], "Database Data.Display Names (for variables)"=w264:string[], "Database Data.SQL Server Info"=w277:T15, "Database Data.Variable Data ID"=w278:string)
        n123 = Concatenate Strings("SELECT * FROM commongui_variables WHERE id ='", w278, "'" ("string")) -> (w258:string)
        n124 = call "SQL Query.vi"("error in (no error)"=w283, "SQL Server Info"=w277, "Query"=w258) -> ("error out"=w282:errorcluster, "data"=w274:string[][])  [unwired: 7 in]
        n125 = Index Array(array=w274) -> (element=w267:string[])  [unwired: 2 in]
        n126 = Array Subset(array=w267, index=9, length=4) -> (w261:string[])
        n127 = Array Subset(array=w267, index=13, length=4) -> (w262:string[])
        n128 = Array Subset(array=w267, index=5, length=4) -> (w263:string[])
        n129 = Build Array(w266, w265, w264, w263, w262, w261) -> (w260:string[][])
        n130 = Transpose 2D Array(2D array=w260) -> (transposed array=w259:string[][])
        n131 = for {
          tunnel: w259 -> [w287] mode=indexing
          tunnel: [w287] -> w280 mode=indexing if=w286
          n132 = call-poly <userlib>:"Filter 1D Array__ogtk.vi"("items to filter"="", "array"=w287) -> ("filtered array"=w289:string[])  [unwired: 4 in, 1 out]
          n133 = Empty Array?(array=w289) -> (empty?=w288:bool)
          n134 = Not(x=w288) -> (.not. x?=w286:bool)
        }
        n135 = Bundle By Name(cluster=w279, "Database Data.Variable display info"=w280) -> (w281:T13)
        n136 = call <vilib>:"Add State(s) to Queue__jki_lib_state_machine.vi"("State(s) in (\"\")"=w285) -> ("States Out"=w284:string)  [unwired: 14 in]
      }
      frame "Data: Initialize Conections" {
        n137 = Unbundle By Name(w296) -> ("Data.Simulate"=w297:bool, "Database Data.Variable display info"=w293:string[][])
        n138 = case shown="False" w297 {
          tunnel: [w303 refnum<k5>[] [] ("Array")] -> w294
          tunnel: w293 -> [w301 _]
          tunnel: [w300 w324] -> w291
          tunnel: w292 -> [w302 w324]
          frame False {
            # "Open TCP Connections"
            n139 = disable-structure shown="Enabled" {
              disable-tunnel: [w319 _] -> w303
              disable-tunnel: w302 -> [w318 _]
              disable-tunnel: w301 -> [w306 w323]
              disable-tunnel: [w305 _] -> w300
              frame Disabled {
                n140 = Build Array (concatenate)(string[][] [["device", "variablename", "defaultvalue", "startvalue", "endvalue"]] ("Data"), w306) -> (w307:string[][])
                "appended array" <- w307
                n141 = call "preset SQL Queries.vi"("error in (no error)"=w318, "Preset Query"=Preset_Query_Enum."Get all devices basic properties") -> ("error out"=w305:errorcluster, "data"=w316:string[][])  [unwired: 7 in, 1 out]
                "Device Infor from Database" <- w316
                n142 = call "scan data to receive to subscribe commands.vi"("ScanData to receive"=w307) -> ("devices"=w312:string[], "Subscribe commands"=w309:string[])  [unwired: 8 in, 1 out]
                "Subscribe commands" <- w309
                n143 = call "get info from core device data.vi"("devices to get data from"=w312, "All Devices Core Info"=w316) -> ("Ports"=w314:string[], "IP Addresses"=w315:string[])  [unwired: 2 in]
                "IP Addresses of interested  devices" <- w315
                n144 = call "TCP multiple open.vi"("timeout ms (60000)"=1000, "Ports"=w314, "error in 1 (no error)"=w305, "IP Addresses"=w315) -> ("error out"=w310:errorcluster, "Array"=w319:refnum<k5>[])  [unwired: 1 out]
                "error TCP Open" <- w310
                n145 = call "tcp multiple write.vi"("Connection ID array"=w319, "error in 1 (no error)"=w310, "messages to send"=w309, "timeout ms (25000)"=1000) -> ("error out"=→"error TCP  Write":errorcluster)
              }
              frame Enabled {
                n146 = call "general plotter variable display info to tcp subsc info.vi"("Array"=w323) -> ("TCP subscriptions info"=w322:T1)  [unwired: 10 in]
                "TCP subscriptions info" <- w322
                n147 = call "Launch TCP data clients.vi"("TCP subscriptions info"=w322) -> ("StopQueue"=→"StopQueue":refnum<queue>, "DataQueue"=→"DataQueue":refnum<queue>)  [unwired: 9 in]
              }
            }
          }
          frame True {
            # "Simulate Mode"
          }
        }
        n148 = Bundle By Name(cluster=w296, "TCP ports"=w294) -> (w295:T13)
        n149 = call <vilib>:"Add State(s) to Queue__jki_lib_state_machine.vi"("State(s) in (\"\")"=w299) -> ("States Out"=w298:string)  [unwired: 14 in]
      }
      frame "Data: Launch TCP Readers" {
        n150 = Unbundle By Name(w329) -> ("Data.Simulate"=w333:bool, "TCP ports"=w332:refnum<k5>[])
        n151 = case shown="False" w333 {
          tunnel: w332 -> [w338 _]
          tunnel: [w339 w367] -> w330
          tunnel: w331 -> [w340 w367]
          tunnel: w329 -> [w337 w366]
          tunnel: [w336 w366] -> w328
          frame False {
            # "Open TCP Connections"
            n152 = disable-structure shown="Enabled" {
              disable-tunnel: w340 -> [w364 _]
              disable-tunnel: [w363 _] -> w339
              disable-tunnel: w338 -> [w362 _]
              disable-tunnel: w337 -> [w361 w365]
              disable-tunnel: [w360 w365] -> w336
              frame Disabled {
                n153 = call <userlib>:"Tick Count (ms)__ogtk.vi"("error in (no error)"=w364) -> ("error out"=w347:errorcluster, "millisecond timer value"=w343:u32)  [unwired: 9 in]
                n154 = vi-ref "tcp tdms single shot.vi"() -> (w358:refnum<vi>)
                n155 = property class="VI"(reference=w358, error in=w347) -> (error out=w359:errorcluster, "Name"=w357:string)  [unwired: 1 out]
                n156 = Select(t=64 ("options"), s=TRUE, f=0 ("options")) -> (s? t:f=w351:i32)
                n157 = Or(x=256 ("options"), y=w351) -> (x .or. y?=w354:i32)
                n158 = Open VI Reference(type specifier VI Refnum (for type only)=refnum<vi> refnum, vi path=w357, options=w354, error in (no error)=w359) -> (vi reference=w348:refnum<vi>, error out=w350:errorcluster)  [unwired: 2 in]
                n159 = Array Size(array=w362) -> (size(s)=w349:i32)
                n160 = invoke class="VI Interface Type 1" method="Populate Async Call Pool"(reference=w348, error in=w350, "MinimumSize"=w349) -> (reference out=w341:refnum<vi>, error out=w346:errorcluster)  [unwired: 2 in, 3 out]
                n161 = Bundle By Name(cluster=w361, "reference out"=w341) -> (w360:T13)
                n162 = call <userlib>:"Tick Count (ms)__ogtk.vi"("error in (no error)"=w346) -> ("error out"=w363:errorcluster, "millisecond timer value"=w344:u32)  [unwired: 9 in]
                n163 = Subtract(x=w344, y=w343) -> (x-y=→"time to open ref":u32)
              }
              frame Enabled {
              }
            }
          }
          frame True {
            # "Simulate Mode"
          }
        }
        n164 = Bundle By Name(cluster=w328, "Data.Start"=TRUE) -> (w327:T13)
        n165 = call <vilib>:"Add State(s) to Queue__jki_lib_state_machine.vi"("State(s) in (\"\")"=w335) -> ("States Out"=w334:string)  [unwired: 14 in]
      }
      frame "---------- UI ----------" {
        # "Do not put any code in this frame.\n(It is a separator no-op. You can make a copy of this frame to create a new UI frame)"
        n166 = call <vilib>:"Add State(s) to Queue__jki_lib_state_machine.vi"("State(s) in (\"\")"=w371) -> ("States Out"=w370:string)  [unwired: 14 in]
      }
      frame "UI: Initialize" {
        # "Initialize the User Interface, here.\n(this is called automatically, by the Macro: Init)"
        n167 = Unbundle By Name(w372) -> ("GUI controls.Stop"=w377:bool, "GUI controls.Tab Control"=w378:enum32{"Home", "Settings", "Plot", "Save"}, "GUI controls.Settings"=w376:bool, "GUI controls.Home"=w375:bool, "GUI controls.Plot"=w374:bool, "Data.Selected Variables"=w373:string[][])  [unwired: 2 out]
        n168 = property on="Stop" class="Bool"("Visible"=w377) -> ()  [unwired: 2 in, 2 out]
        n169 = property on="Database Variable List" class="MCListbox (strict)"("ItemNames"=w373) -> ()  [unwired: 2 in, 2 out]
        n170 = property on="Settings" class="Bool (strict)"("Value"=w376) -> ()  [unwired: 2 in, 2 out]
        n171 = property on="Plot" class="Bool (strict)"("Value"=w374) -> ()  [unwired: 2 in, 2 out]
        n172 = property on="Home" class="Bool (strict)"("Value"=w375) -> ()  [unwired: 2 in, 2 out]
        n173 = property on="Tab Control" class="TabCtl (strict)"("Value"=w378) -> ()  [unwired: 2 in, 2 out]
        n174 = call <vilib>:"Add State(s) to Queue__jki_lib_state_machine.vi"("State(s) in (\"\")"=w381) -> ("States Out"=w380:string)  [unwired: 14 in]
      }
      frame "UI: Cursor Set" {
        # "Argument"
        # "Set and Unset Cursor Busy.\n(Usage: \"UI: Cursor Set >> Busy|Idle\")"
        n175 = case shown="\"Idle\", Default" w382 {
          tunnel: w384 -> [w389 w391]
          tunnel: [w388 w390] -> w383
          frame "Idle", Default {
            n176 = call <vilib>:"Unset Busy.vi"("error in (no error)"=w389) -> ("error out"=w388:errorcluster)  [unwired: 10 in]
          }
          frame "Busy" {
            n177 = call <vilib>:"Set Busy.vi"("error in (no error)"=w391) -> ("error out"=w390:errorcluster)  [unwired: 9 in, 1 out]
          }
        }
        n178 = call <vilib>:"Add State(s) to Queue__jki_lib_state_machine.vi"("State(s) in (\"\")"=w387) -> ("States Out"=w386:string)  [unwired: 14 in]
      }
      frame "UI: Front Panel State" {
        # "Argument"
        # "Set Front Panel Open or Closed\n(Usage: \"UI: Front Panel State >> Open|Close\")"
        n179 = Unbundle By Name(w394) -> ("Core.Current VI Reference"=w393:refnum<vi>)
        n180 = case shown="\"Open\", Default" w392 {
          tunnel: w396 -> [w402 w415]
          tunnel: [w404 w416] -> w395
          tunnel: w393 -> [w403 w413]
          frame "Open", Default {
            n181 = property class="VI"(reference=w403, error in=w402) -> (reference out=w400:refnum<vi>, error out=w401:errorcluster, "Front Panel.Open"=w399:bool)
            n182 = case shown="True" w399 {
              tunnel: [w407 w410] -> w404
              tunnel: w401 -> [w406 w410]
              tunnel: w400 -> [w405 _]
              frame False {
                n183 = invoke class="VI" method="FP.Open"(reference=w405, error in=w406, "Activate"=TRUE, "State"=T7."Standard") -> (error out=w407:errorcluster)  [unwired: 1 in, 4 out]
              }
              frame True {
              }
            }
          }
          frame "Close" {
            n184 = property class="VI"(reference=w413, error in=w415) -> (reference out=w412:refnum<vi>, error out=w414:errorcluster, "Front Panel.Open"=w411:bool)
            n185 = case shown="True" w411 {
              tunnel: [w417 w420] -> w416
              tunnel: w414 -> [w417 w419]
              tunnel: w412 -> [_ w418]
              frame False {
              }
              frame True {
                n186 = invoke class="VI" method="FP.Close"(reference=w418, error in=w419) -> (error out=w420:errorcluster)  [unwired: 1 in, 2 out]
              }
            }
          }
        }
        n187 = call <vilib>:"Add State(s) to Queue__jki_lib_state_machine.vi"("State(s) in (\"\")"=w398) -> ("States Out"=w397:string)  [unwired: 14 in]
      }
      frame "---------- Macro ----------" {
        # "Do not put any code in this frame.\n(It is a separator no-op. You can make a copy of this frame to create a new Macro frame)"
        n188 = call <vilib>:"Add State(s) to Queue__jki_lib_state_machine.vi"("State(s) in (\"\")"=w424) -> ("States Out"=w423:string)  [unwired: 14 in]
      }
      frame "Macro: Initialize" {
        # "Initialization Macro\n(This is called once, when the VI starts)"
        n189 = call <userlib>:"Fit VI window to Largest Dec__ogtk.vi"("error in (no error)"=w429, "border spacing (2 px)"=0) -> ("error out"=w428:errorcluster)  [unwired: 4 in, 1 out]
        n190 = call <vilib>:"Add State(s) to Queue__jki_lib_state_machine.vi"("State(s) in Front (\"\")"="Data: Initialize\nInitialize Core Data\nUI: Initialize\nUI: Front Panel State >> Open\nData: Read Database\nData: Read Database 2\nData: Initialize Conections\nData: Launch TCP Readers\nAction: Select All Data", "State(s) in (\"\")"=w431) -> ("States Out"=w430:string)  [unwired: 13 in]
      }
      frame "Macro: Exit" {
        # "Exit Macro\n(This is called once, when the VI exits)"
        n191 = Unbundle By Name(w438) -> ("Core.Close Panel on Exit?"=w437:bool)
        n192 = Select(t="UI: Front Panel State >> Close", s=w437, f="") -> (s? t:f=w434:string)
        n193 = call <vilib>:"Add State(s) to Queue__jki_lib_state_machine.vi"("State(s) in (\"\")"=w434, "State(s) at Back (\"\")"="Data: Cleanup\nExit") -> ("States Out"=w432:string)  [unwired: 13 in]
        n194 = call <vilib>:"Add State(s) to Queue__jki_lib_state_machine.vi"("State(s) in Front (\"\")"=w432, "State(s) in (\"\")"=w441) -> ("States Out"=w440:string)  [unwired: 13 in]
      }
      frame "---------- Action ----------" {
        # "Template Separator\n(You can make a copy of, or modify, this frame)"
        n195 = call <vilib>:"Add State(s) to Queue__jki_lib_state_machine.vi"("State(s) in (\"\")"=w445) -> ("States Out"=w444:string)  [unwired: 14 in]
      }
      frame "Action: Start Plotting" {
        n196 = property on="Stop" class="Bool"("Visible"=TRUE) -> ()  [unwired: 2 in, 2 out]
        n197 = Unbundle By Name(w451) -> ("Data.Selected Variables"=w455:string[][])
        n198 = Array Size(array=w455) -> (size(s)=w456:i32[])
        n199 = Index Array(array=w456) -> (element=w453:i32)  [unwired: 1 in]
        n200 = Add(x=w453, y=w453) -> (x+y=w452:i32)
        n201 = Initialize Array(cluster{timestamp[], dbl[]} {[], []} ("Graph i"), w452) -> (w446:cluster{timestamp[], dbl[]}[])
        n202 = Bundle By Name(cluster=w451, "Data.No of Selected Variables"=w452, "Graph.Graph Data Long"=w446, "Graph.Graph Data Short"=w446) -> (w450:T13)
        n203 = call <vilib>:"Add State(s) to Queue__jki_lib_state_machine.vi"("State(s) in (\"\")"=w449) -> ("States Out"=w448:string)  [unwired: 14 in]
      }
      frame "Action: Plot Data" {
        # "Timer calculations:\nPlot 1 data updates \nafter every 30 seconds"
        # "#TODO Hide the RHS scales on the long term plot and the\nLHS scales on the short term plot\nBring both plots closer. - Completed Priyanka"
        # "This case is used for long term and short term data plotting"
        n204 = Unbundle By Name(w476) -> ("Graph.ms timer value"=w463:u32, "Graph.Graph Data Long"=w474:T16, "Data.Data"=w472:dbl[], "Data.Selected Variables"=w458:string[][], "Data.Currently selected items"=w478:i32[], "Graph.Long term plot"=w459:refnum<vi>, "Graph.Graph Data Short"=w460:T16)
        n205 = First Call?() -> (First Call?: T/F=w468:bool)
        n206 = call <userlib>:"Tick Count (ms)__ogtk.vi"() -> ("millisecond timer value"=w464:u32)  [unwired: 10 in, 1 out]
        n207 = Not(x=w468) -> (.not. x?=w466:bool)
        n208 = Subtract(x=w464, y=w463) -> (x-y=w469:u32)
        n209 = call "Plot.vi"("dev-Var data"=w472, "Selected Variables"=w458, "Currently selected items"=w478) -> ("Plot Data"=w471:dbl[])  [unwired: 12 in]
        n210 = Greater Or Equal?(x=w469, y=u32 30000 ("min time between updates")) -> (x >= y?=w467:bool)
        n211 = And(x=w467, y=w466) -> (x .and. y?=w465:bool)
        n212 = call "Graph Properties Runtime.vi"("Long Term Graph"=w459, "Selected Variables"=w458, "Plot Data"=w471) -> ()  [unwired: 12 in, 1 out]
        n213 = case shown="True" w465 {
          tunnel: "Clear Graph" -> [_ w495]
          tunnel: w474 -> [w489 w493]
          tunnel: [w489 w492] -> w473
          tunnel: w471 -> [_ w491]
          tunnel: w464 -> [_ w490]
          tunnel: w463 -> [w488 _]
          tunnel: [w488 w490] -> w462
          frame False {
          }
          frame True {
            n214 = call "Long Term PLot.vi"("Graph Data"=w493, "Plot Data"=w491, "Clear Graph"=w495, "Max Number of Datapoints"=2000.0) -> ("Graph Data 2"=w492:T16)  [unwired: 11 in]
            "Long Term Plot" <- w492
          }
        }
        n215 = case shown="True" w466 {
          tunnel: "Clear Graph" -> [_ w487]
          tunnel: w460 -> [w482 w485]
          tunnel: w471 -> [_ w484]
          tunnel: [w482 w483] -> w461
          frame False {
          }
          frame True {
            n216 = call "Long Term PLot.vi"("Graph Data"=w485, "Plot Data"=w484, "Clear Graph"=w487, "Max Number of Datapoints"=500.0) -> ("Graph Data 2"=w483:T16)  [unwired: 11 in]
            "short Term Plot" <- w483
          }
        }
        n217 = Bundle By Name(cluster=w476, "Graph.ms timer value"=w462, "Graph.Graph Data Long"=w473, "Graph.Graph Data Short"=w461) -> (w477:T13)
        n218 = call <vilib>:"Add State(s) to Queue__jki_lib_state_machine.vi"("State(s) in (\"\")"=w481) -> ("States Out"=w480:string)  [unwired: 14 in]
      }
      frame "Action: Collect Data" {
        # "Collect Data from TCP port/ Simulated data"
        n219 = Unbundle By Name(w501) -> ("Data.Selected Variables"=w496:string[][], "Data.Simulate"=w505:bool, "TCP ports"=w504:refnum<k5>[], "reference out"=w498:refnum<vi>)
        n220 = case shown="False" w505 {
          tunnel: w504 -> [w512 _]
          tunnel: w503 -> [w508 w535]
          tunnel: [w508 w535] -> w502
          tunnel: [w509 w530] -> w499
          tunnel: w498 -> [w511 w534]
          tunnel: [w510 w534] -> w497
          tunnel: w496 -> [_ w532]
          frame False {
            # "Data from TCP port"
            n221 = disable-structure shown="Enabled" {
              disable-tunnel: w512 -> [w525 _]
              disable-tunnel: w511 -> [w523 _]
              disable-tunnel: [w520 _] -> w510
              disable-tunnel: [w514 w526] -> w509
              frame Disabled {
                n222 = call "multi tcp tdms single shot no open.vi"("TCP connections"=w525, "timeout ms"=6000, "type specifier VI Refnum (for type only)"=w523) -> ("type specifier out"=w520:refnum<vi>, "Output"=w524:T17, "error out 2"=→"error out":errorcluster)  [unwired: 1 in, 2 out]
                n223 = Unbundle By Name(w524) -> ("tcp Data parsed array"=w521:string[][])
                n224 = Index Array(array=w521, index (row)=1 ("disabled index (col)")) -> (element=w516:string[])  [unwired: 1 in]
                "Data read by TCP" <- w516
                n225 = Delete From Array(array=w516, length=1, index=0) -> (array with subset deleted=w515:string[])  [unwired: 1 out]
                n226 = Fract/Exp String To Number(string=w515) -> (number=w514:dbl[])  [unwired: 3 in, 1 out]
              }
              frame Enabled {
                n227 = local read "TCP subscriptions info"() -> (w529:T1)
                n228 = local read "DataQueue"() -> (w528:refnum<queue>)
                n229 = call "tcp data queue to requested values.vi"("TCP subscriptions info"=w529, "Queue in"=w528) -> ("Array"=w527:string[])  [unwired: 7 in, 2 out]
                n230 = Fract/Exp String To Number(string=w527) -> (number=w526:dbl[])  [unwired: 3 in, 1 out]
              }
            }
          }
          frame True {
            # "Simulated Data"
            n231 = Index Array(array=w532, index (col)=3 ("disabled index (col)")) -> (element=w531:string[])  [unwired: 1 in]
            n232 = for {
              tunnel: w531 -> [w538] mode=indexing
              tunnel: [w536] -> w530 mode=indexing
              n233 = Fract/Exp String To Number(string=w538) -> (number=w537:dbl)  [unwired: 3 in, 1 out]
              n234 = Random Number (0-1)() -> (number: 0 to 1=w539:dbl)
              n235 = Add(x=w539, y=w537) -> (x+y=w536:dbl)
            }
          }
        }
        n236 = Bundle By Name(cluster=w501, "Data.Data"=w499, "reference out"=w497) -> (w500:T13)
        n237 = call <vilib>:"Add State(s) to Queue__jki_lib_state_machine.vi"("State(s) in (\"\")"=w507) -> ("States Out"=w506:string)  [unwired: 14 in]
      }
      frame "Action: Select All Data" {
        # "Graph properties needs to set only once \nso coded here"
        # "Select variables from configuration file"
        n238 = Unbundle By Name(w553) -> ("Database Data.Variable display info"=w544:string[][], "Graph.Long term plot"=w552:refnum<vi>, "Graph.Short term plot"=w551:refnum<vi>)
        n239 = Array Size(array=w544) -> (size(s)=w548:i32[])
        n240 = Build Array(w552, w551) -> (w550:refnum<vi>[])
        n241 = Index Array(array=w548) -> (element=w547:i32)  [unwired: 1 in]
        n242 = Empty Array?(array=w544) -> (empty?=w540:bool)
        n243 = property on="Database Variable List" class="MCListbox (strict)"(error in=w541, "ItemNames"=w544) -> (error out=w542:errorcluster)  [unwired: 1 in, 1 out]
        n244 = case shown="False" w540 {
          tunnel: w550 -> [w562 _]
          tunnel: [w561 w563] -> w549
          tunnel: [w560 _] -> w546
          tunnel: w541 -> [w559 w563]
          tunnel: w544 -> [w558 _]
          frame False {
            n245 = call "Set Graph Properties.vi"("error out 2"=w559, "Selected Variables"=w558, "Reference Array"=w562) -> ("error out"=w561:errorcluster, "Legend rows"=w560:i32)  [unwired: 7 in]
          }
          frame True {
          }
        }
        n246 = for {
          N: w547 -> [_]
          tunnel: [w564] -> w554 mode=indexing
          i -> [w564]
        }
        n247 = control-ref of="Database Variable List"() -> (w543:refnum<vi>)
        n248 = Bundle By Name(cluster=w553, "Data.Currently selected items"=w554, "Data.Selected Variables"=w544, "Data.Legend Rows"=w546) -> (w555:T13)
        n249 = call "Listbox Properties.vi"("error in (no error)"=w542, "Configuration File Variable List 2"=w543) -> ()  [unwired: 9 in, 1 out]
        n250 = call <vilib>:"Add State(s) to Queue__jki_lib_state_machine.vi"("State(s) in Front (\"\")"="Action: Start Plotting" ("State(s) in Front (\"\")"), "State(s) in (\"\")"=w557) -> ("States Out"=w556:string)  [unwired: 13 in]
      }
    }
  }
